vi "sort all.vi"(0 "Get All Control Values Variant":cluster{"Name":string, "Variant Data":variant}[](array[cluster])) -> (1 "output":T1(array[cluster]), 2 "Values":sgl[](array[numeric]))   [LabVIEW 2016, in "flat top.lvlib"]
doc: "This vi sorts all through all of the controls of a vi and only selects the ones that can be flat topped"
uses:
  flat top.lvlib
panel:
  out "error out":errorcluster
  in  "error in":errorcluster
  in  "control":cluster{"String":string, "value":dbl}
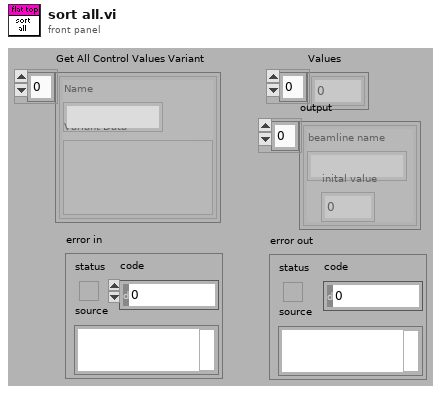
[diagram p1: front panel]
types:
  T1 = cluster{"beamline name":string, "inital value":dbl}[]
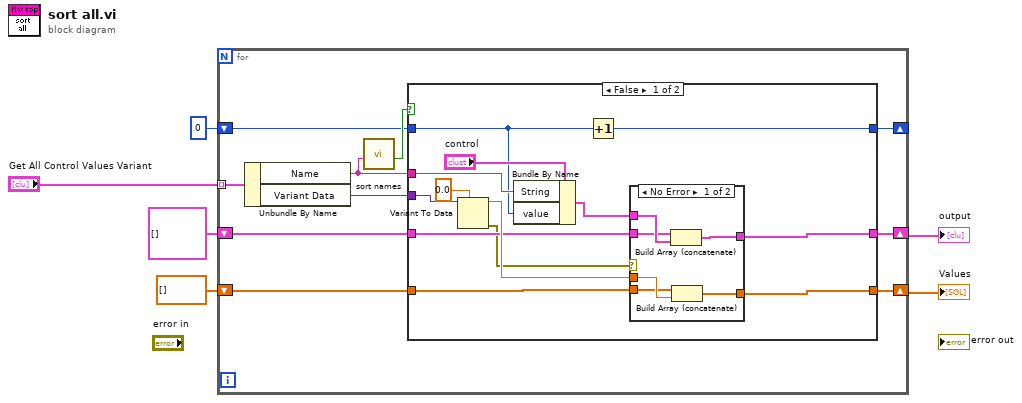
[diagram p0: block diagram]
diagram:
  n1 = for {
    tunnel: "Get All Control Values Variant" -> [w16] mode=indexing
    shift-right: [w15] -> w5
    shift-left: cluster{"String":string, "value":dbl}[] [] -> [w14]
    shift-right: [w10] -> w6
    shift-left: sgl[] [] -> [w9]
    shift-right: [w7] -> _
    shift-left: 0 -> [w8]
    n2 = Unbundle By Name(w16) -> ("Name"=w13:string, "Variant Data"=w12:variant)
    n3 = call "sort names.vi"("Name"=w13) -> ("display value?"=w11:bool)  [unwired: 9 in, 1 out]
    n4 = case shown="False" w11 {
      tunnel: [w19 w40] -> w15
      tunnel: w14 -> [w18 w40]
      tunnel: w13 -> [w22 _]
      tunnel: w12 -> [w29 _]
      tunnel: [w26 w39] -> w10
      tunnel: w9 -> [w25 w39]
      tunnel: [w24 w38] -> w7
      tunnel: w8 -> [w21 w38]
      frame False {
        n5 = Variant To Data(type=sgl 0.0, Variant=w29) -> (data=w27:sgl, error out=w17:errorcluster)  [unwired: 1 in]
        n6 = Bundle By Name(cluster="control", "String"=w22, "value"=w21) -> (w20:cluster{"String":string, "value":dbl})
        n7 = Increment(x=w21) -> (x+1=w24:i32)
        n8 = case shown="No Error" w17 {
          tunnel: w27 -> [w35 _]
          tunnel: [w34 w36] -> w26
          tunnel: w25 -> [w33 w36]
          tunnel: w20 -> [w32 _]
          tunnel: [w31 w37] -> w19
          tunnel: w18 -> [w30 w37]
          frame No Error {
            n9 = Build Array (concatenate)(w30, w32) -> (w31:cluster{"String":string, "value":dbl}[])
            n10 = Build Array (concatenate)(w33, w35) -> (w34:sgl[])
          }
          frame Error {
          }
        }
      }
      frame True {
      }
    }
  }
  "Values" <- w6
  "output" <- w5
